vi "Get - Time Data OBJ State.vi"(0 "reference in":refnum<class "WaveFile.lvclass">, 5 "error in (no error)":errorcluster) -> (13 "New Time Data Obj?":bool, 14 "reference out":refnum<class "WaveFile.lvclass">, 19 "error out":errorcluster)   [LabVIEW 2022 SP3, in "WaveFile.lvclass"]
uses:
  WaveFile.lvclass
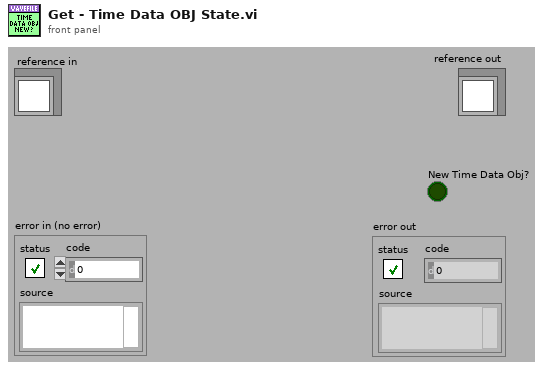
[diagram p1: front panel]
types:
  T1 = typedef "WaveFile.lvclass/ObjectAttributes.ctl" = cluster{"Time Data":refnum<class "GSwFormDSP.lvclass">, "New Time Data Obj?":bool, "NIST File Header":T2}
  T2 = typedef "WaveFile.lvclass/NIST File Header.ctl" = cluster{"Version":string, "Header Nb Bytes":i32, "Nb Samples":i32, "Nb Bytes/sample":i32, "Nb Channels":i32, "byte order":enum16{"big-endian, network order", "native, host order", "little-endian"}, "Fs":dbl, "Valid Header?":bool}
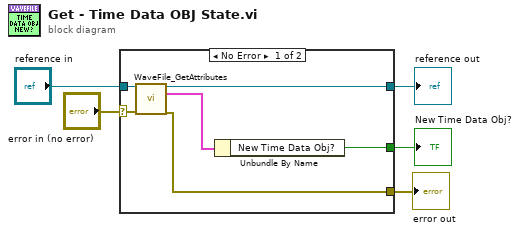
[diagram p0: block diagram]
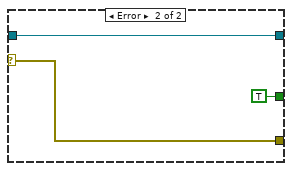
[diagram p2: hidden frame]
diagram:
  n1 = case shown="No Error" "error in (no error)" {
    selector: "error in (no error)" -> [w11 w14]
    tunnel: [w10 w14] -> w4
    tunnel: [w9 w13] -> w2
    tunnel: "reference in" -> [w7 w13]
    tunnel: [w6 TRUE ("New Time Data Obj?")] -> w1
    frame No Error {
      n2 = call "WaveFile_GetAttributes.vi"("reference in"=w7, "error in (no error)"=w11) -> ("reference out"=w9:refnum<class "WaveFile.lvclass">, "attributes"=w8:T1, "error out"=w10:errorcluster)  [unwired: 14 in, 1 out]
      n3 = Unbundle By Name(w8) -> ("New Time Data Obj?"=w6:bool)
    }
    frame Error {
    }
  }
  "error out" <- w4
  "reference out" <- w2
  "New Time Data Obj?" <- w1
